vi "INTERLOCK SETTING.vi"() -> ()   [LabVIEW 2017]
uses:
  <vilib>/addons/database/Connection.llb/DB Tools Open Connec (Path).vi
  <vilib>/addons/database/NI_Database_API.lvlib
panel:
  in  "table":string[][](table)
  in  "EXIT":bool
  in  "SAVE":bool
  # "PARAMETERS VALUE"
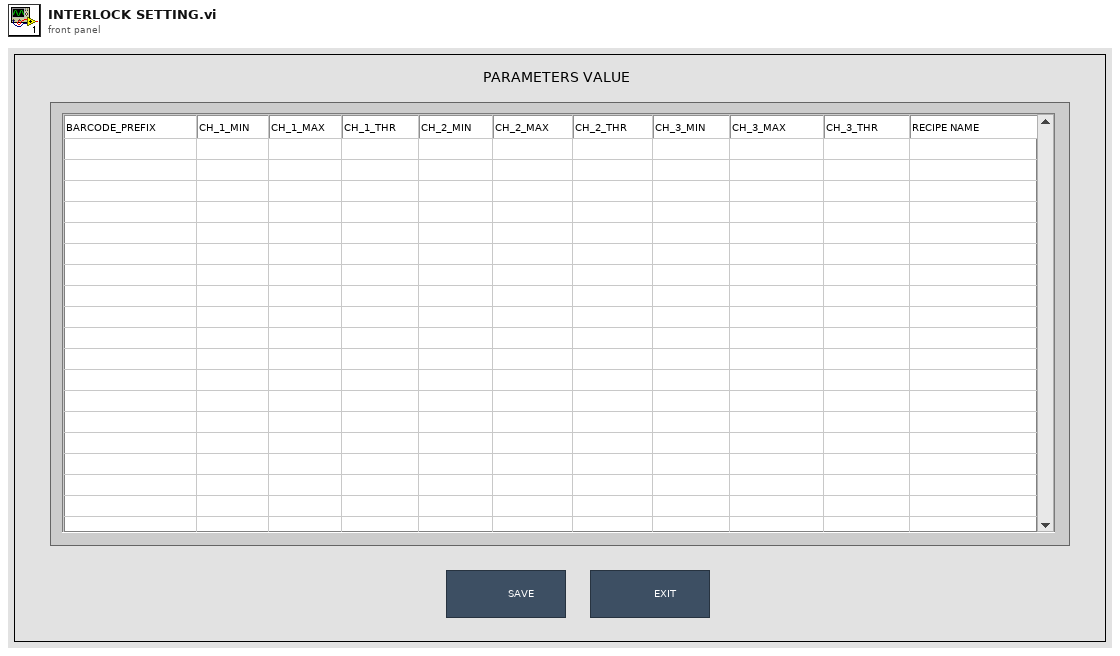
[diagram p1: front panel]
types:
  T1 = typedef "NI_Database_API.lvlib/Conn ObjectReference.ctl" = refnum<k1>
  T2 = cluster{"table":string[], "table":string[], "table":string[], "table":string[], "table":string[], "table":string[], "table":string[], "table":string[], "table":string[], "table":string[], "table":string[]}
  T3 = enum32{"invalid app kind", "Development System", "Run Time System", "Student Edition", "Embedded LabVIEW", "Evaluation", "Custom"}
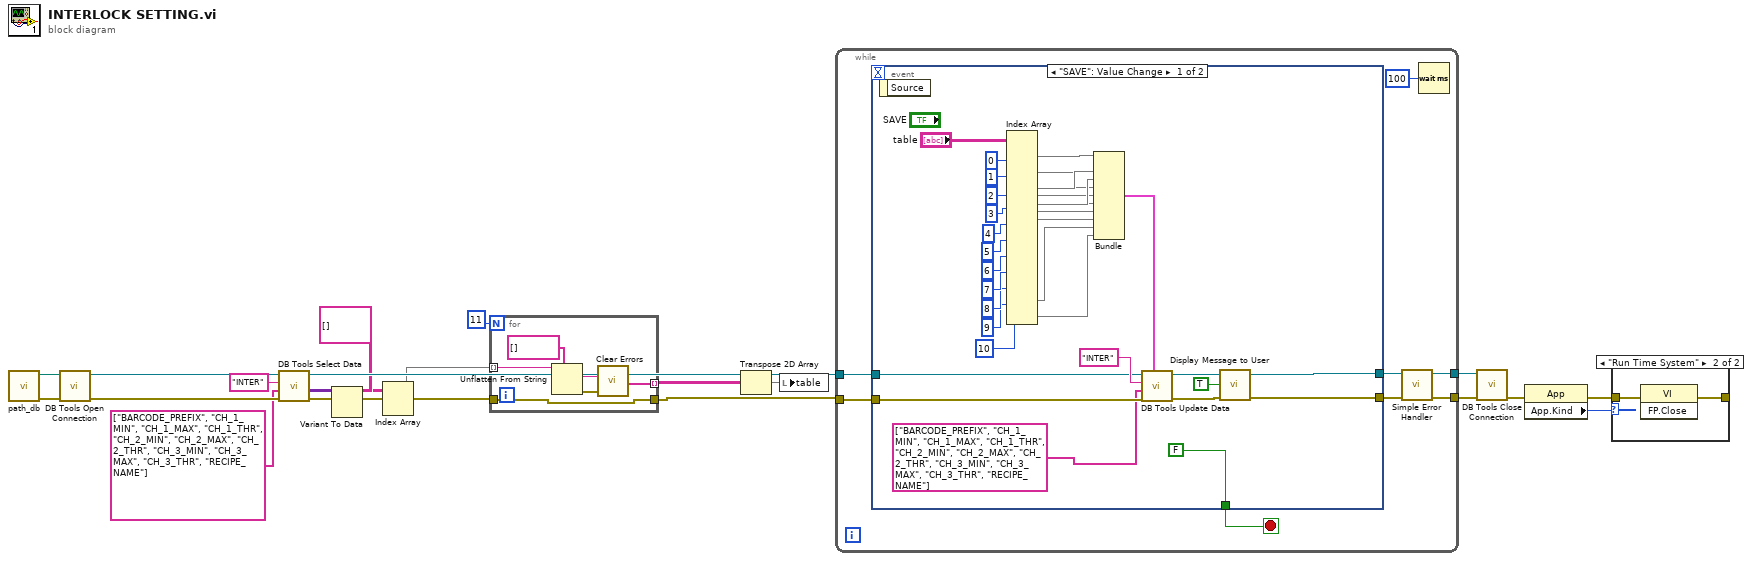
[diagram p0: block diagram]
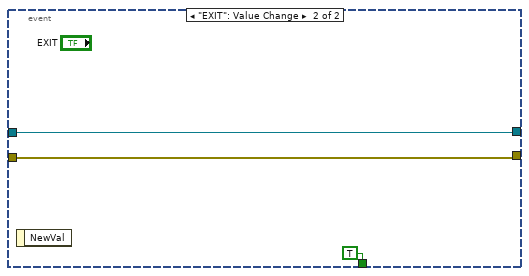
[diagram p3: hidden frame]
diagram:
  n1 = call "path_db.vi"() -> ("error out"=w8:errorcluster, "resulting string"=w7:path)  [unwired: 10 in]
  n2 = call-poly <vilib>:"DB Tools Open Connection.vi"("error in (no error)"=w8, "connection information"=w7) -> ("error out"=w14:errorcluster, "connection reference"=w16:T1)  [unwired: 6 in]
  n3 = call <vilib>:"DB Tools Select Data.vi"("error in (no error)"=w14, "columns"=string[] ["BARCODE_PREFIX", "CH_1_MIN", "CH_1_MAX", "CH_1_THR", "CH_2_MIN", "CH_2_MAX", "CH_2_THR", "CH_3_MIN", "CH_3_MAX", "CH_3_THR", "RECIPE_NAME"], "table"="INTER", "connection reference"=w16) -> ("error out"=w2:errorcluster, "data"=w11:variant[][], "connection reference out"=w15:T1)  [unwired: 2 in]
  n4 = Variant To Data(type=string[][] [], Variant=w11) -> (data=w10:string[][])  [unwired: 1 in, 1 out]
  n5 = Index Array(array=w10) -> (element=w4:string[])  [unwired: 2 in]
  n6 = for {
    N: 11 -> [_]
    tunnel: w4 -> [w25] mode=indexing
    tunnel: [w23] -> w3 mode=indexing
    tunnel: w2 -> [w22]
    tunnel: [w22] -> w1
    n7 = Unflatten From String(type=string[] [], binary string=w25) -> (value=w23:string[], error out=w26:errorcluster)  [unwired: 3 in, 1 out]
    n8 = call <vilib>:"Clear Errors.vi"("error in (no error)"=w26) -> ()  [unwired: 5 in, 2 out]
  }
  n9 = Transpose 2D Array(2D array=w3) -> (transposed array=w9:string[][])
  n10 = local write "table"(w9) -> ()
  n11 = while {
    tunnel: w1 -> [w32]
    tunnel: w15 -> [w31]
    tunnel: [w30] -> w21
    tunnel: [w28] -> w20
    stop <- w33 stop-if-true
    n12 = event shown="[0] \"SAVE\": Value Change" {
      selector: _ -> [_ _]
      dyn-events: _ -> [_ _]
      timeout: _ -> [_ _]
      tunnel: [FALSE TRUE] -> w33
      tunnel: w32 -> [w64 w67]
      tunnel: w31 -> [w63 w68]
      tunnel: [w62 w68] -> w30
      tunnel: [w37 w67] -> w29
      event "SAVE": Value Change {
        n13 = event-data() -> ()  [unwired: 1 in, 1 out]
        n14 = Index Array(array="table", index (col) #1=0 ("disabled index (col)"), index (col) #2=1 ("index (col)"), index (col) #3=2 ("index (col)"), index (col) #4=3 ("index (col)"), index (col) #5=4 ("index (col)"), index (col) #6=5 ("index (col)"), index (col) #7=6 ("index (col)"), index (col) #8=7 ("index (col)"), index (col) #9=8 ("index (col)"), index (col) #10=9 ("index (col)"), index (col) #11=10 ("index (col)")) -> (element #1=w56:string[], element #2=w53:string[], element #3=w54:string[], element #4=w55:string[], element #5=w44:string[], element #6=w43:string[], element #7=w42:string[], element #8=w41:string[], element #9=w40:string[], element #10=w39:string[], element #11=w34:string[])  [unwired: 11 in]
        n15 = Bundle("table"=w56, "table"=w53, "table"=w54, "table"=w55, "table"=w44, "table"=w43, "table"=w42, "table"=w41, "table"=w40, "table"=w39, "table"=w34) -> (w52:T2)  [unwired: 1 in]
        n16 = call <vilib>:"DB Tools Update Data.vi"("data"=w52, "error in (no error)"=w64, "columns"=string[] ["BARCODE_PREFIX", "CH_1_MIN", "CH_1_MAX", "CH_1_THR", "CH_2_MIN", "CH_2_MAX", "CH_2_THR", "CH_3_MIN", "CH_3_MAX", "CH_3_THR", "RECIPE_NAME"], "table"="INTER", "connection reference"=w63) -> ("error out"=w38:errorcluster, "connection reference out"=w62:T1)  [unwired: 5 in]
        n17 = call "Display Message to User"("error in (no error)"=w38, "Enable"=TRUE) -> ("error out"=w37:errorcluster)  [unwired: 8 in, 1 out]
      }
      event "EXIT": Value Change {
        n18 = event-data() -> ()  [unwired: 1 in, 1 out]
      }
    }
    n19 = call <vilib>:"Simple Error Handler.vi"("error in (no error)"=w29) -> ("error out"=w28:errorcluster)  [unwired: 4 in, 4 out]
    n20 = Wait (ms)(milliseconds to wait=u32 100) -> ()  [unwired: 1 out]
  }
  n21 = call <vilib>:"DB Tools Close Connection.vi"("error in (no error)"=w20, "connection reference"=w21) -> ("error out"=w17:errorcluster)  [unwired: 5 in]
  n22 = property class="App"(error in=w17) -> (error out=w18:errorcluster, "App.Kind"=w19:T3)  [unwired: 1 in, 1 out]
  n23 = case shown="\"Run Time System\"" w19 {
    tunnel: w18 -> [w70 w72]
    tunnel: [w70 w71] -> _
    frame Default {
    }
    frame "Run Time System" {
      n24 = invoke class="VI" method="FP.Close"(error in=w72) -> (error out=w71:errorcluster)  [unwired: 2 in, 2 out]
    }
  }
